vi "Compute Whiskers.vi"(7 "ORIGINAL ARRAY":dbl[](array[numeric]) format="%.2f") -> (2 "min":dbl, 3 "max":dbl)   [LabVIEW 2022 SP3, in "Box Plots.lvlib"]
doc: "Calculates the begining and end points of the upper and lower whiskers."
uses:
  Box Plots.lvlib
panel:
  in  "error in (no error)":errorcluster
  out "Numeric":i32
  out "SORTED ARRAY OUT":dbl[](array[numeric])
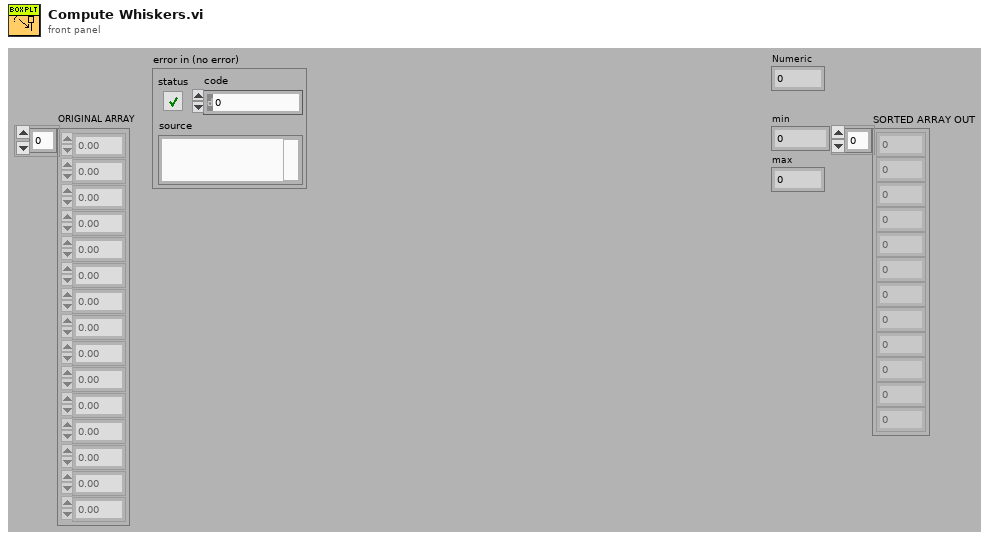
[diagram p1: front panel]
types:
  T1 = cluster{"DBL VALUE":dbl, "POSITION OF VAL":i32}[]
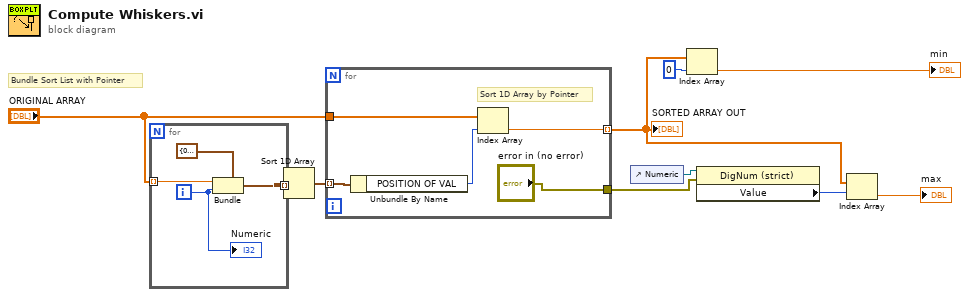
[diagram p0: block diagram]
diagram:
  # "Bundle Sort List with Pointer"
  n1 = for {
    tunnel: "ORIGINAL ARRAY" -> [w14] mode=indexing
    tunnel: [w13] -> w9 mode=indexing
    i -> [w11]
    n2 = Bundle(cluster=cluster{"DBL VALUE":dbl, "POSITION OF VAL":i32} {"DBL VALUE"=0.0, "POSITION OF VAL"=0}, "DBL VALUE"=w14, "POSITION OF VAL"=w11) -> (w13:cluster{"DBL VALUE":dbl, "POSITION OF VAL":i32})
    "Numeric" <- w11
  }
  n3 = Sort 1D Array(array=w9) -> (sorted array=w10:T1)
  n4 = for {
    tunnel: "ORIGINAL ARRAY" -> [w19]
    tunnel: [w18] -> w5 mode=indexing
    tunnel: w10 -> [w17] mode=indexing
    tunnel: ["error in (no error)"] -> w2
    # "Sort 1D Array by Pointer"
    n5 = Unbundle By Name(w17) -> ("POSITION OF VAL"=w16:i32)
    n6 = Index Array(array=w19, index=w16) -> (element=w18:dbl)
  }
  "SORTED ARRAY OUT" <- w5
  n7 = control-ref of="Numeric"() -> (w3:refnum<vi>)
  n8 = Index Array(array=w5, index=0) -> (element=→"min":dbl)
  n9 = property class="DigNum (strict)"(reference=w3, error in=w2) -> ("Value"=w1:i32)  [unwired: 2 out]
  n10 = Index Array(array=w5, index=w1) -> (element=→"max":dbl)
